vi "gentec-M-Link.Find err string.vi"(1 "string":string) -> (0 "Found":bool)   [LabVIEW 2014, in "gentec-M-Link - Driver.lvlib"]
doc: "This VI sets the incoming string to upercase characters and searches for \"ERR\"."
uses:
  gentec-M-Link - Driver.lvlib
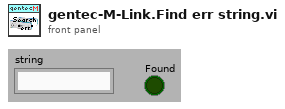
[diagram p1: front panel]
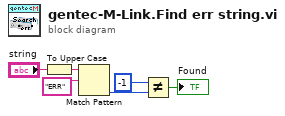
[diagram p0: block diagram]
diagram:
  n1 = To Upper Case(1:"string") -> (0:w2:string)
  n2 = Match Pattern(string=w2, regular expression="ERR") -> (offset past match=w6:i32)  [unwired: 1 in, 3 out]
  n3 = Not Equal?(x=-1, y=w6) -> (x != y?=→"Found":bool)
